vi "Query current delay position.vi"(8 "error in (no error)":errorcluster, 9 "Unit":enum16{"fs", "ps", "um", "mm", "counts"}(ring), 10 "Delay Line":enum16{"K1", "K2", "K3"}(ring), 11 "Query delay position":bool) -> (0 "error out":errorcluster, 3 "Current delay position (optical path)":string)   [LabVIEW 2009]
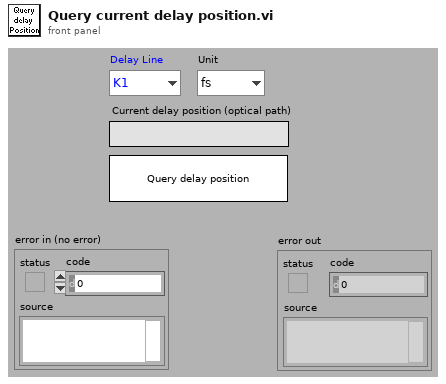
[diagram p1: front panel]
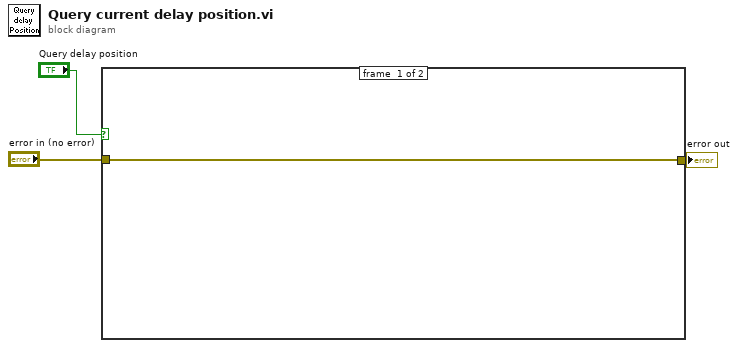
[diagram p0: block diagram]
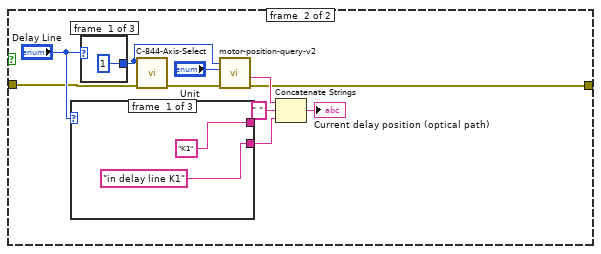
[diagram p2: hidden frame]
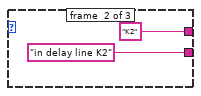
[diagram p3: hidden frame]
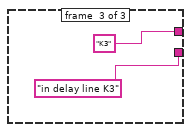
[diagram p4: hidden frame]
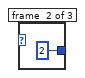
[diagram p5: hidden frame]
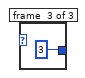
[diagram p6: hidden frame]
diagram:
  n1 = case shown="True" "Query delay position" {
    tunnel: "error in (no error)" -> [w4 w6]
    tunnel: [w4 w5] -> w1
    frame #0 {
    }
    frame #1 {
      n2 = case shown="\"K2\", Default" "Delay Line" {
        tunnel: ["in delay line K1" "in delay line K2" "in delay line K3"] -> w11
        tunnel: ["K1" "K2" "K3"] -> _
        frame #0 {
        }
        frame #1 {
        }
        frame #2 {
        }
      }
      n3 = case shown="\"K3\"" "Delay Line" {
        tunnel: [u8 1 u8 2 u8 3] -> w8
        frame #0 {
        }
        frame #1 {
        }
        frame #2 {
        }
      }
      n4 = call "C-844-Axis-Select.vi"("error in (no error)"=w6, "Axis Select"=w8) -> ("error out"=w14:errorcluster)  [unwired: 8 in, 1 out]
      n5 = call "motor-position-query-v2.vi"("error in (no error)"=w14, "Unit"="Unit", "Axis Select"=w8) -> ("error out"=w5:errorcluster, "Initial Position of motor"=w10:string)  [unwired: 5 in, 2 out]
      n6 = Concatenate Strings(w10, " ", w11) -> (→"Current delay position (optical path)":string)
    }
  }
  "error out" <- w1
